vi "SetEnumValueByString.vi"(3 "error in (no error)":errorcluster, 4 "strValue":string, 5 "strName":string, 6 "nInputHandle":u64) -> (0 "error out":errorcluster, 1 "GX_STATUS":i32, 2 "nOutputHandle":u64)   [LabVIEW 2016, in "GxLVLib.lvlib"]
uses:
  GxLVLib.lvlib
  GxIAPI.dll
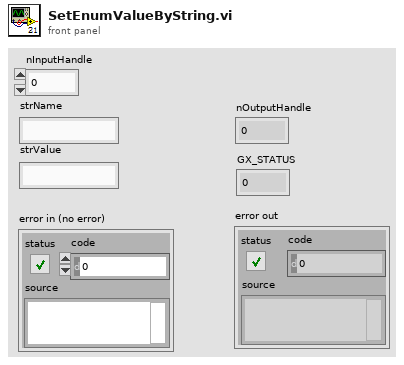
[diagram p1: front panel]
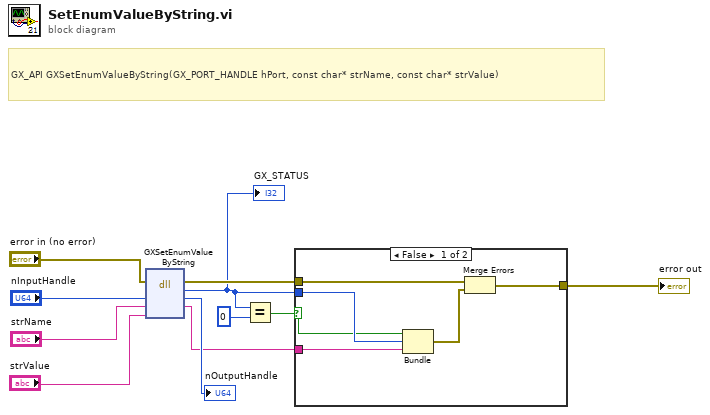
[diagram p0: block diagram]
diagram:
  # "GX_API GXSetEnumValueByString(GX_PORT_HANDLE hPort, const char* strName, const char* strValue)"
  n1 = dll-call lib="GxIAPI.dll" fn="GXSetEnumValueByString"(error in="error in (no error)", "phDevice"="nInputHandle", "strName"="strName", "strValue"="strValue") -> (error out=w10:errorcluster, "GX_STATUS"=w4:i32, "phDevice"=→"nOutputHandle":i64, "strName"=w7:string)  [unwired: 3 in, 1 out]
  "GX_STATUS" <- w4
  n2 = Equal?(x=w4, y=0) -> (x = y?=w9:bool)
  n3 = case shown="False" w9 {
    selector: w9 -> [w13 _]
    tunnel: w10 -> [w17 w18]
    tunnel: [w16 w18] -> w5
    tunnel: w4 -> [w14 _]
    tunnel: w7 -> [w12 _]
    frame False {
      n4 = Bundle(w13, "GX_STATUS"=w14, "strName"=w12) -> (w15:cluster{bool, "GX_STATUS":i32, "strName":string})  [unwired: 1 in]
      n5 = Merge Errors(w17, w15) -> (w16:errorcluster)
    }
    frame True {
    }
  }
  "error out" <- w5
